vi "Volume Descriptor.vi"(8 "error in (no error)":errorcluster, 11 "VGS_VolumeDescriptor in":refnum<class "VGS_VolumeDescriptor.lvclass">) -> (0 "error out":errorcluster, 3 "VGS_VolumeDescriptor out":refnum<class "VGS_VolumeDescriptor.lvclass">)   [LabVIEW 2022 SP3, in "LV_VGS.lvlib" / "VGS_VolumeDescriptor.lvclass"]
uses:
  VGS_VolumeDescriptor.lvclass
  VGS_VolumeDescriptor.lvclass/VGS_VolumeDescriptor.ctl
  C:/Users/Andrey/Documents/GitHub/LV_VGS/vgs_project.dll
  vgs_project.dll
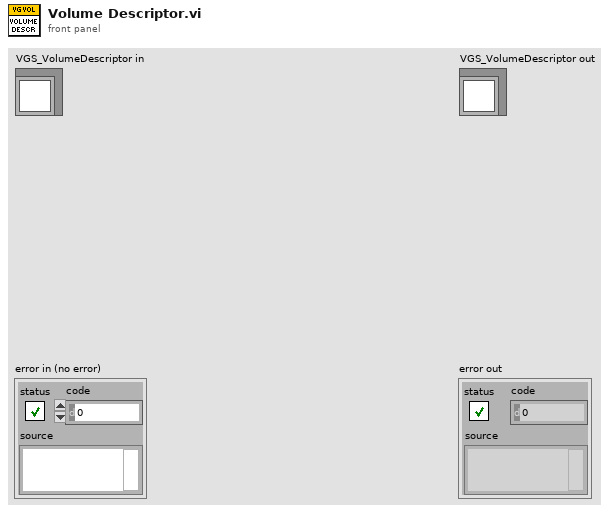
[diagram p1: front panel]
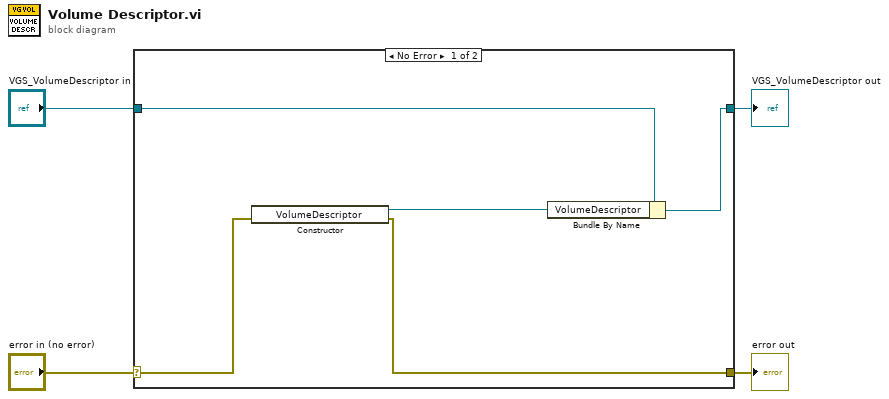
[diagram p0: block diagram]
diagram:
  n1 = case shown="No Error" "error in (no error)" {
    selector: "error in (no error)" -> [w6 w11]
    tunnel: [w5 w11] -> w3
    tunnel: [w8 w10] -> w1
    tunnel: "VGS_VolumeDescriptor in" -> [w9 w10]
    frame No Error {
      n2 = constructor class="VolumeDescriptor"(error in=w6) -> (reference out=w7:refnum<k24>, error out=w5:errorcluster)  [unwired: 2 in, 1 out]
      n3 = Bundle By Name(cluster=w9, "VolumeDescriptor"=w7) -> (w8:refnum<class "VGS_VolumeDescriptor.lvclass">)
    }
    frame Error {
    }
  }
  "error out" <- w3
  "VGS_VolumeDescriptor out" <- w1
